vi "Dpc Open Jtag.vi"(0 "phif":u32, 5 "szdvc":string, 7 "perc":i32, 9 "ptrid":u16, 11 "error in (no error)":errorcluster) -> (3 "function return":i32, 4 "phif out":u32, 6 "szdvc out":string, 8 "perc out":i32, 10 "ptrid out":u16, 15 "error out":errorcluster)   [LabVIEW 2011, in "LVH-Adept.lvlib" / "DPCUTIL.lvlib"]
doc: "DPCAPI BOOL DpcOpenJtag(HANDLE * phif, char * szdvc, ERC * perc, TRID * ptrid);"
uses:
  DPCUTIL.lvlib
  Resources/dpcutil.dll
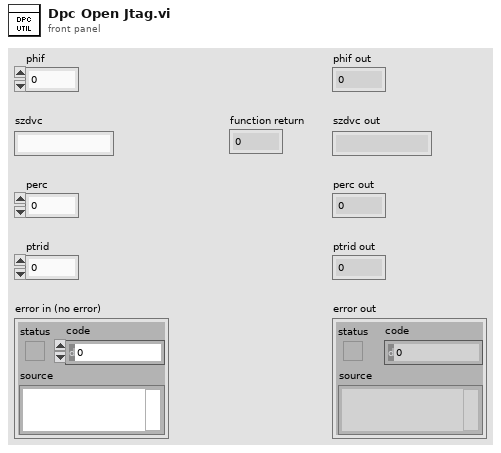
[diagram p1: front panel]
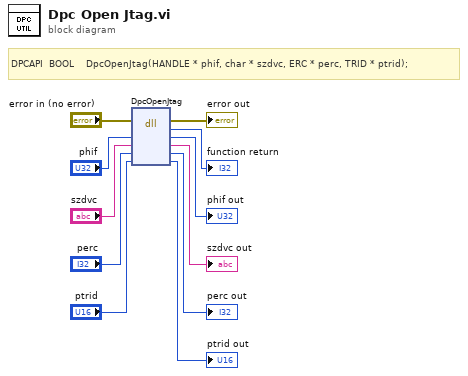
[diagram p0: block diagram]
diagram:
  # "DPCAPI  BOOL    DpcOpenJtag(HANDLE * phif, char * szdvc, ERC * perc, TRID * ptrid);"
  n1 = dll-call lib="C:/github/labviewhacker/LVH-Adept/LabVIEW/vi.lib/LabVIEW Hacker/Adept/Private/Resources/dpcutil.*" fn="DpcOpenJtag"(error in="error in (no error)", "phif"="phif", "szdvc"="szdvc", "perc"="perc", "ptrid"="ptrid") -> (error out=→"error out":errorcluster, →"function return":i32, "phif"=→"phif out":u32, "szdvc"=→"szdvc out":string, "perc"=→"perc out":i32, "ptrid"=→"ptrid out":u16)  [unwired: 2 in, 1 out]
